vi "FSM_new.vi"() -> ()   [LabVIEW 2016]
panel:
  out "Current target":dbl[](array[numeric])
  out "note":string
  out "Waveform Graph 2":dbl[](graph)
  out "Select traing signal":i32
  out "Saved Target":dbl[][](array[numeric])
  out "Number of Signals":i32
  out "Signal Captured":dbl[][](array[numeric])
  in  "Signal Capture":bool
  out "Error_out":dbl[](array[numeric])
  out "Final Error":dbl
  out "Waveform Graph":dbl[](graph)
  in  "Inference":bool
  in  "Training":bool
  out "Enum":T1(ring)
  out "Weights_oX":dbl[][](array[numeric])
  out "Weights_hX":dbl[][](array[numeric])
  out "Outputs_oX":dbl[](array[numeric])
  out "Outputs_hX":dbl[](array[numeric])
  in  "Target 6":dbl
  in  "Target 5":dbl
  in  "Target 7":dbl
  in  "Target 8":dbl
  in  "Learning rate":dbl
  in  "Offset 2":dbl
  in  "Offset 1":dbl
  out "Random values generated":bool
  out "Training end":bool
  in  "A+E+F":dbl
  in  "A+B+D":dbl
  in  "C+Ch+B":dbl
  in  "C+E+G":dbl
  in  "Stop":bool
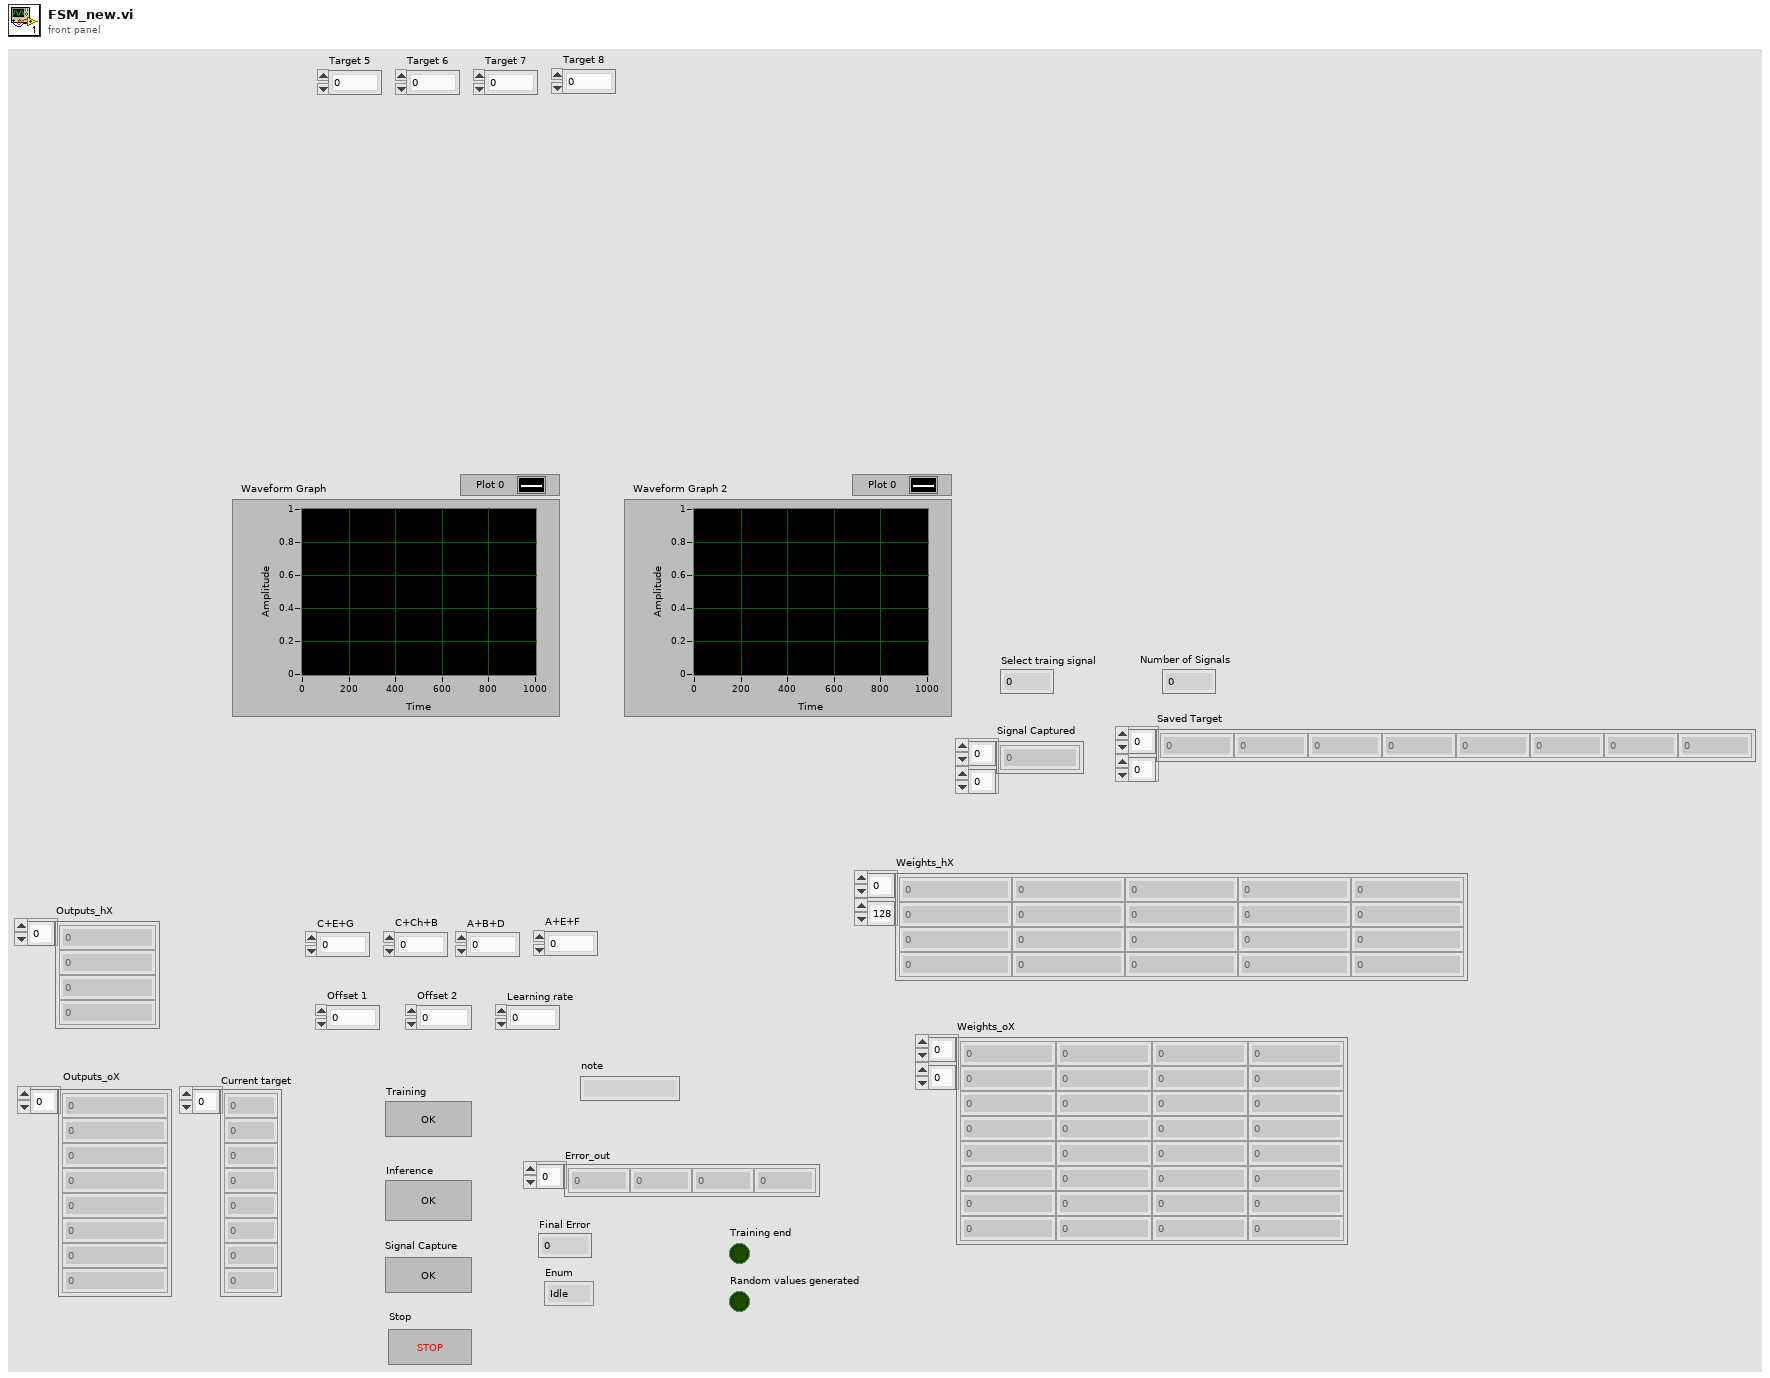
[diagram p1: front panel]
types:
  T1 = enum16{"Idle", "Generate weights", "Training mode", "Inference mode"}
  T2 = enum16{"Idle", "Generate weights", "Training mode", "Inference mode", "Signal Capture"}
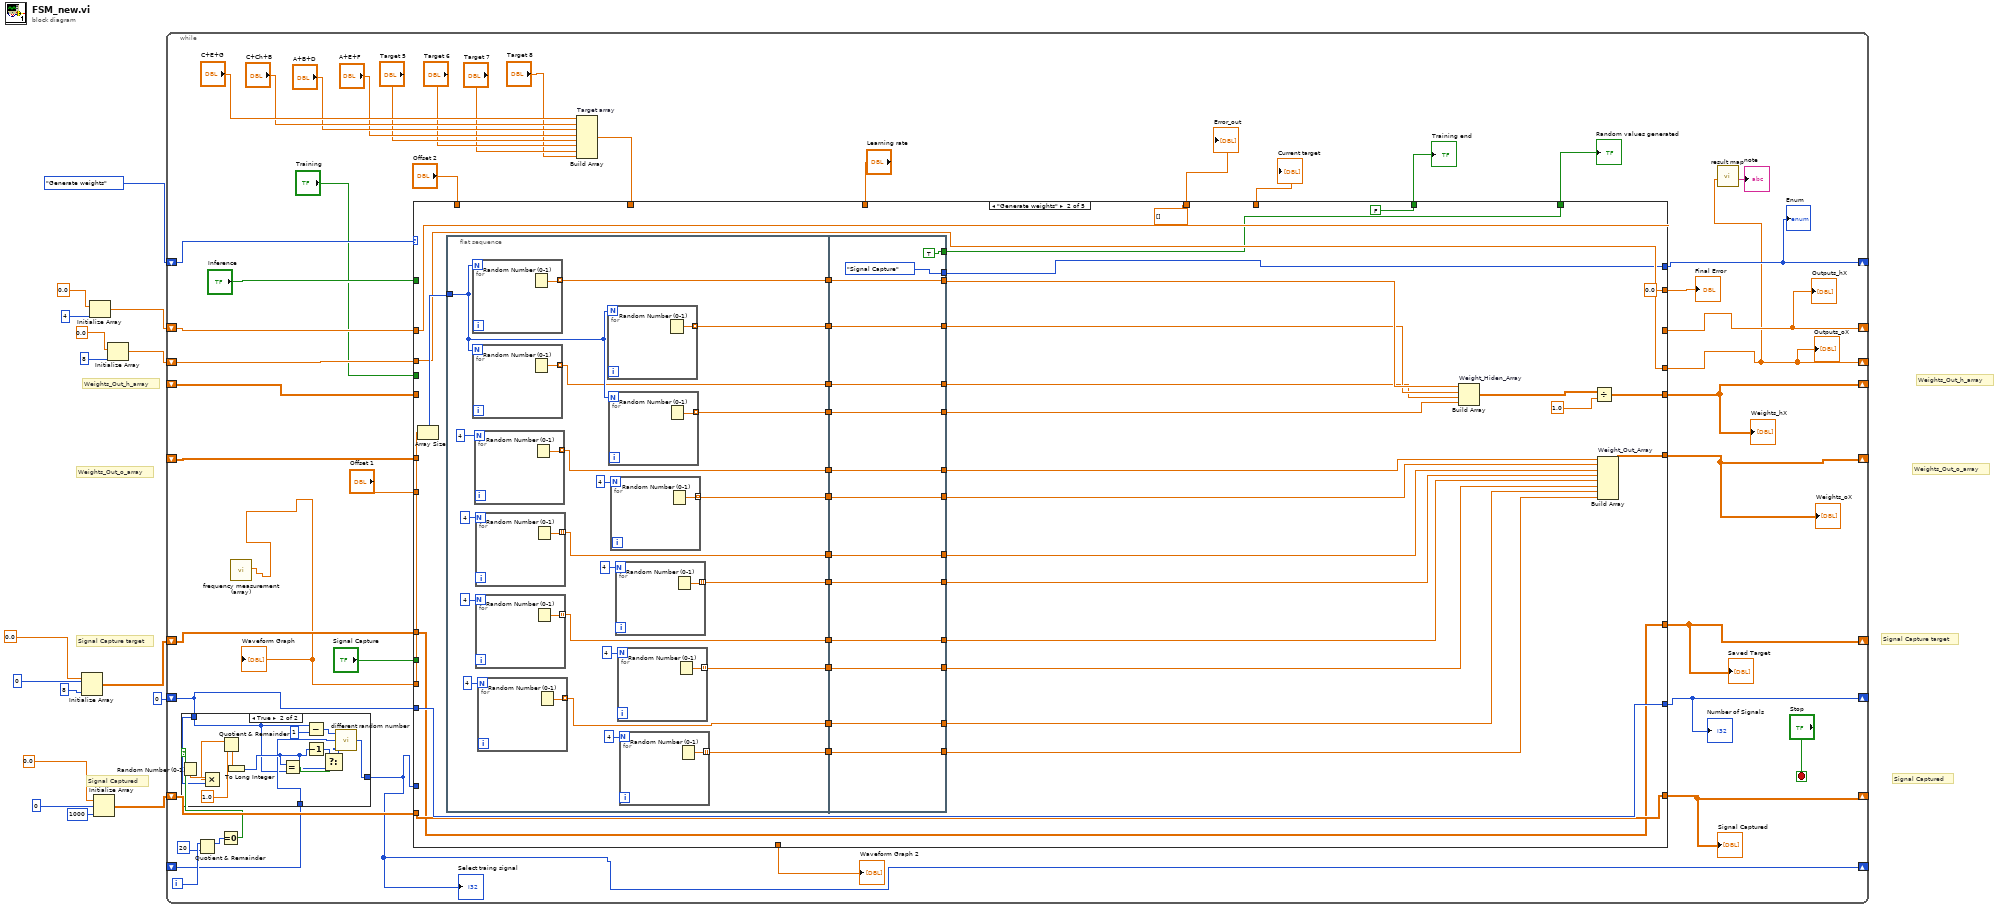
[diagram p0: block diagram]
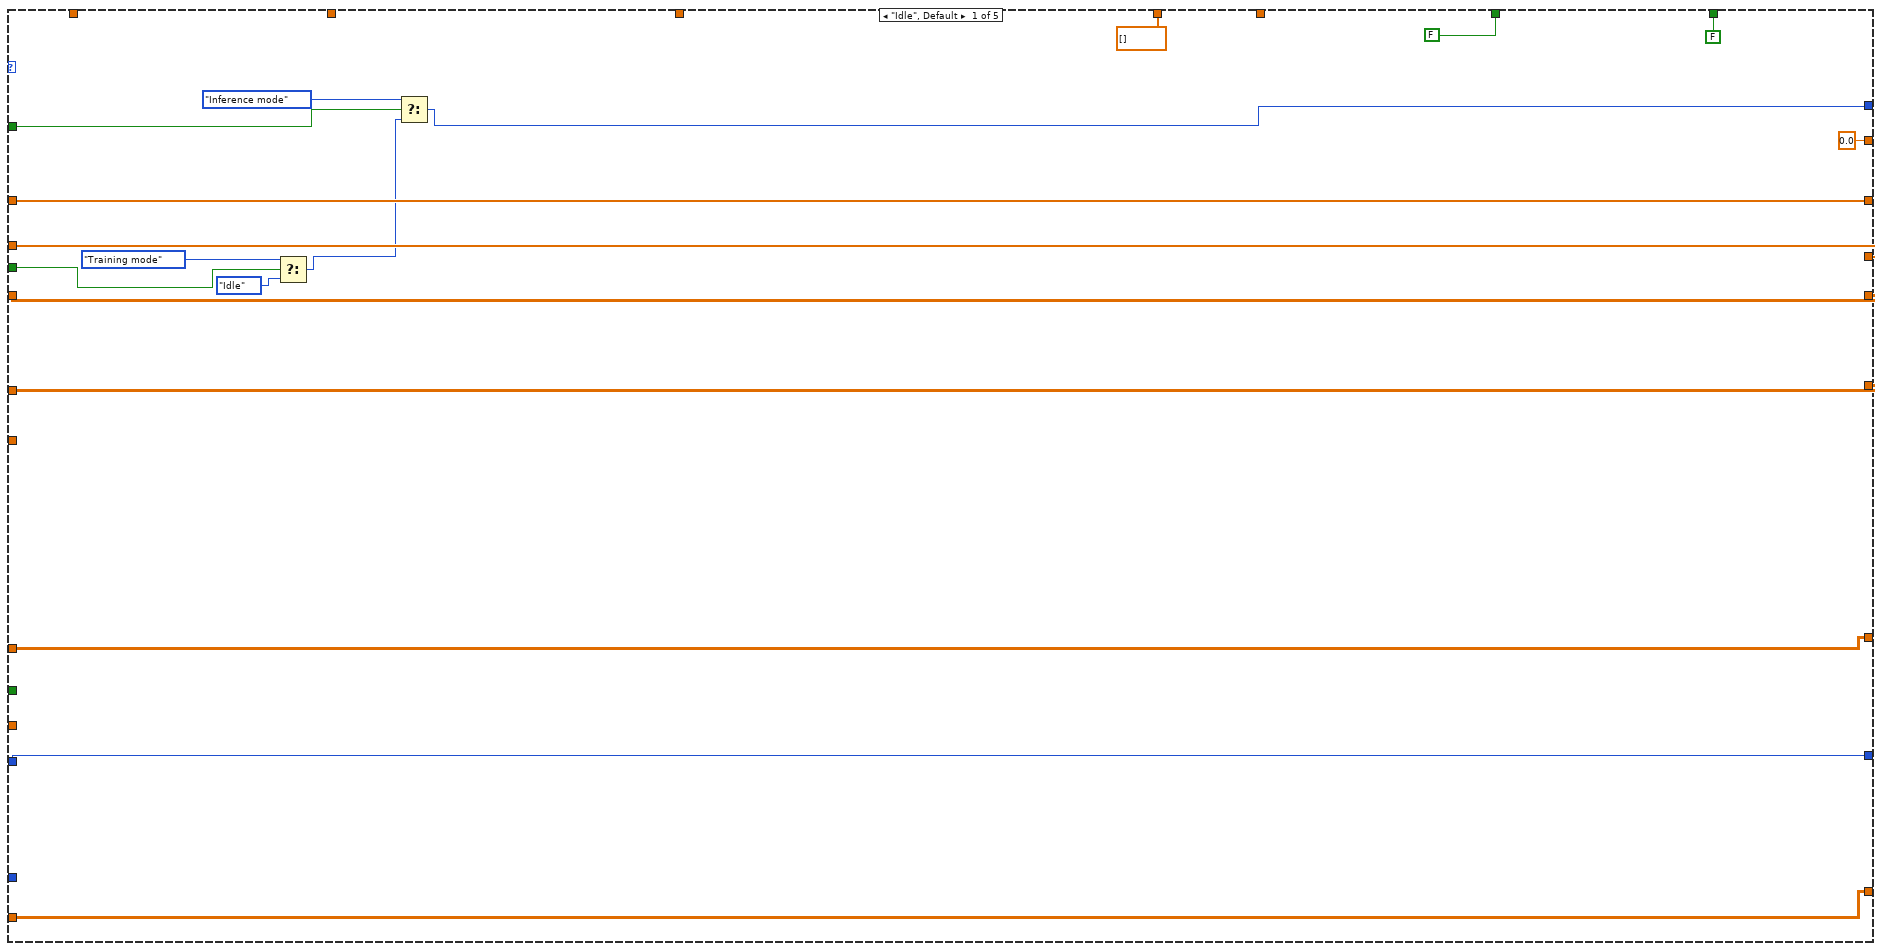
[diagram p3: hidden frame]
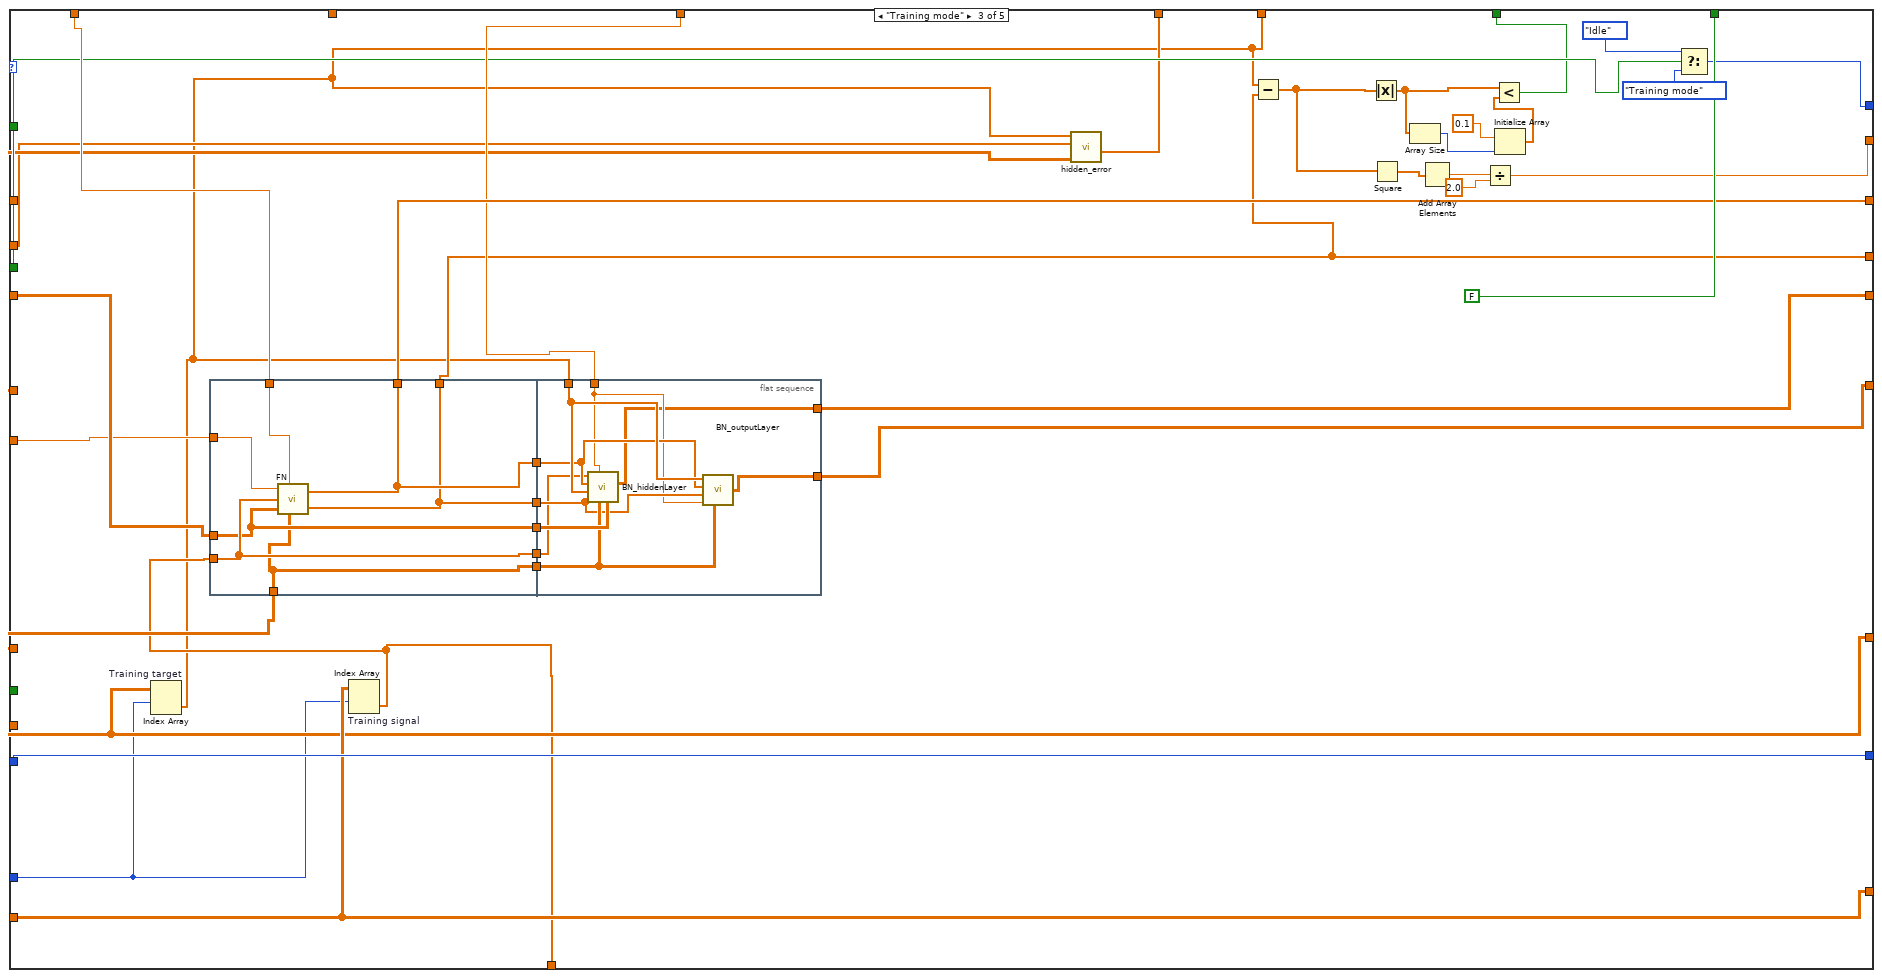
[diagram p4: hidden frame]
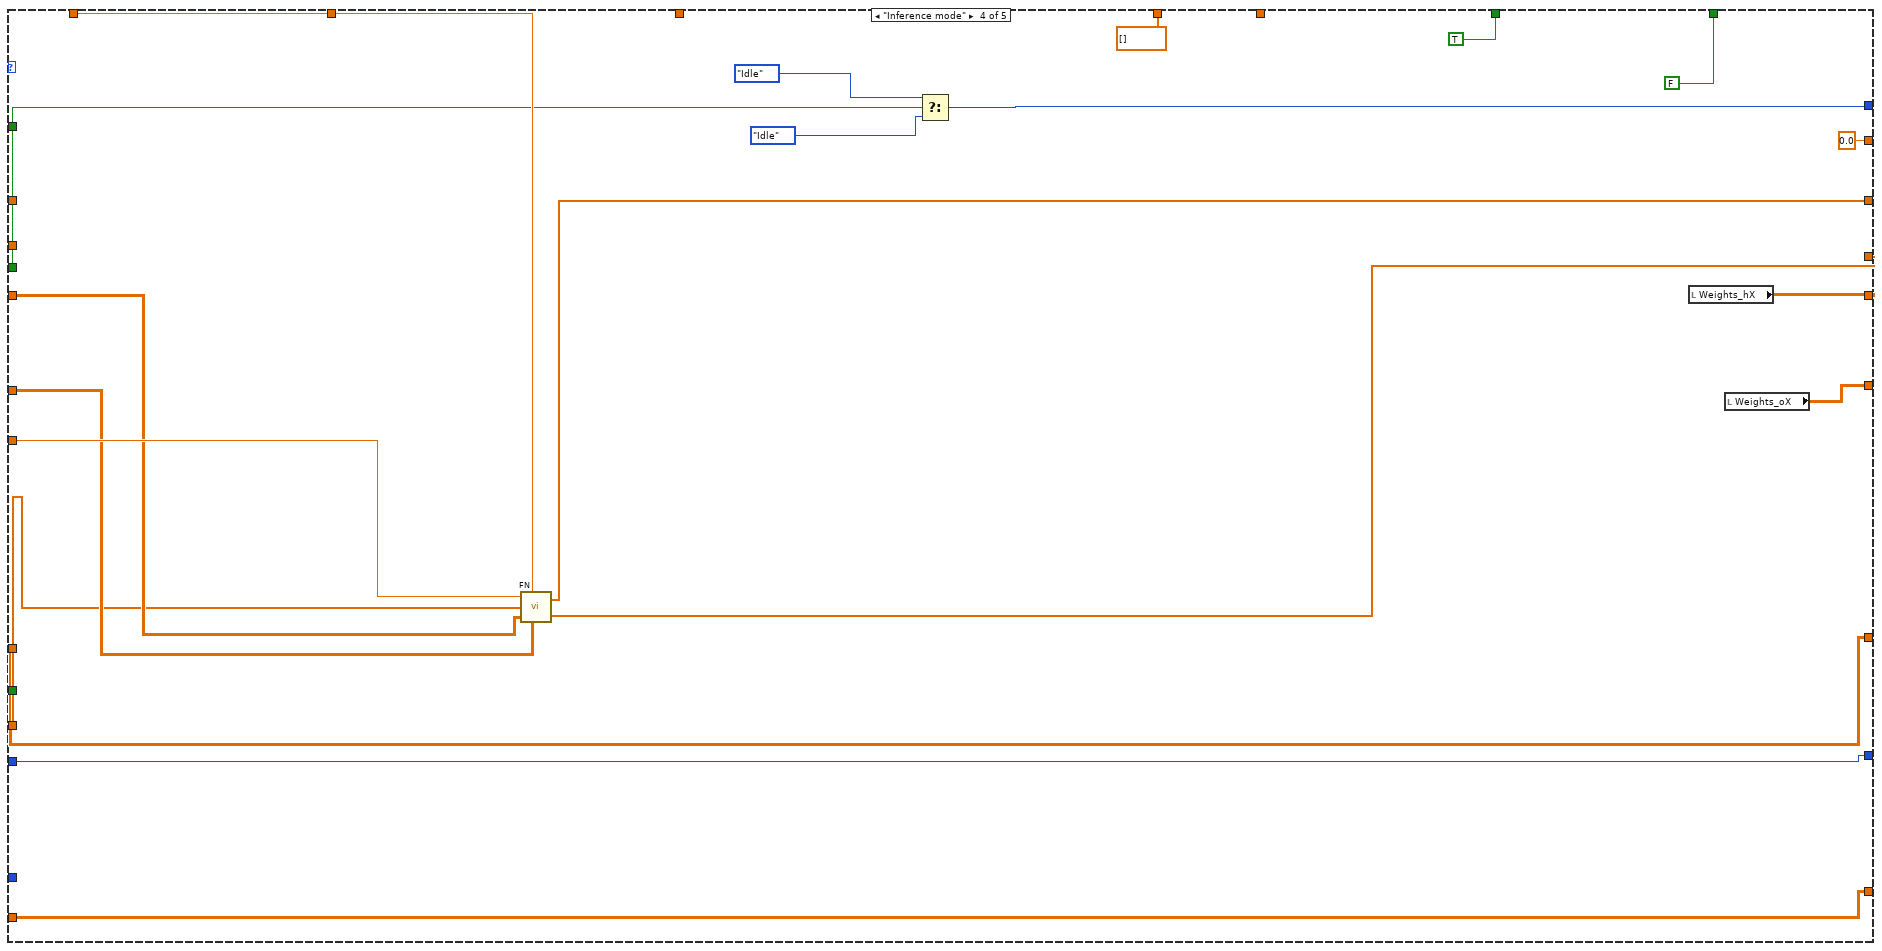
[diagram p5: hidden frame]
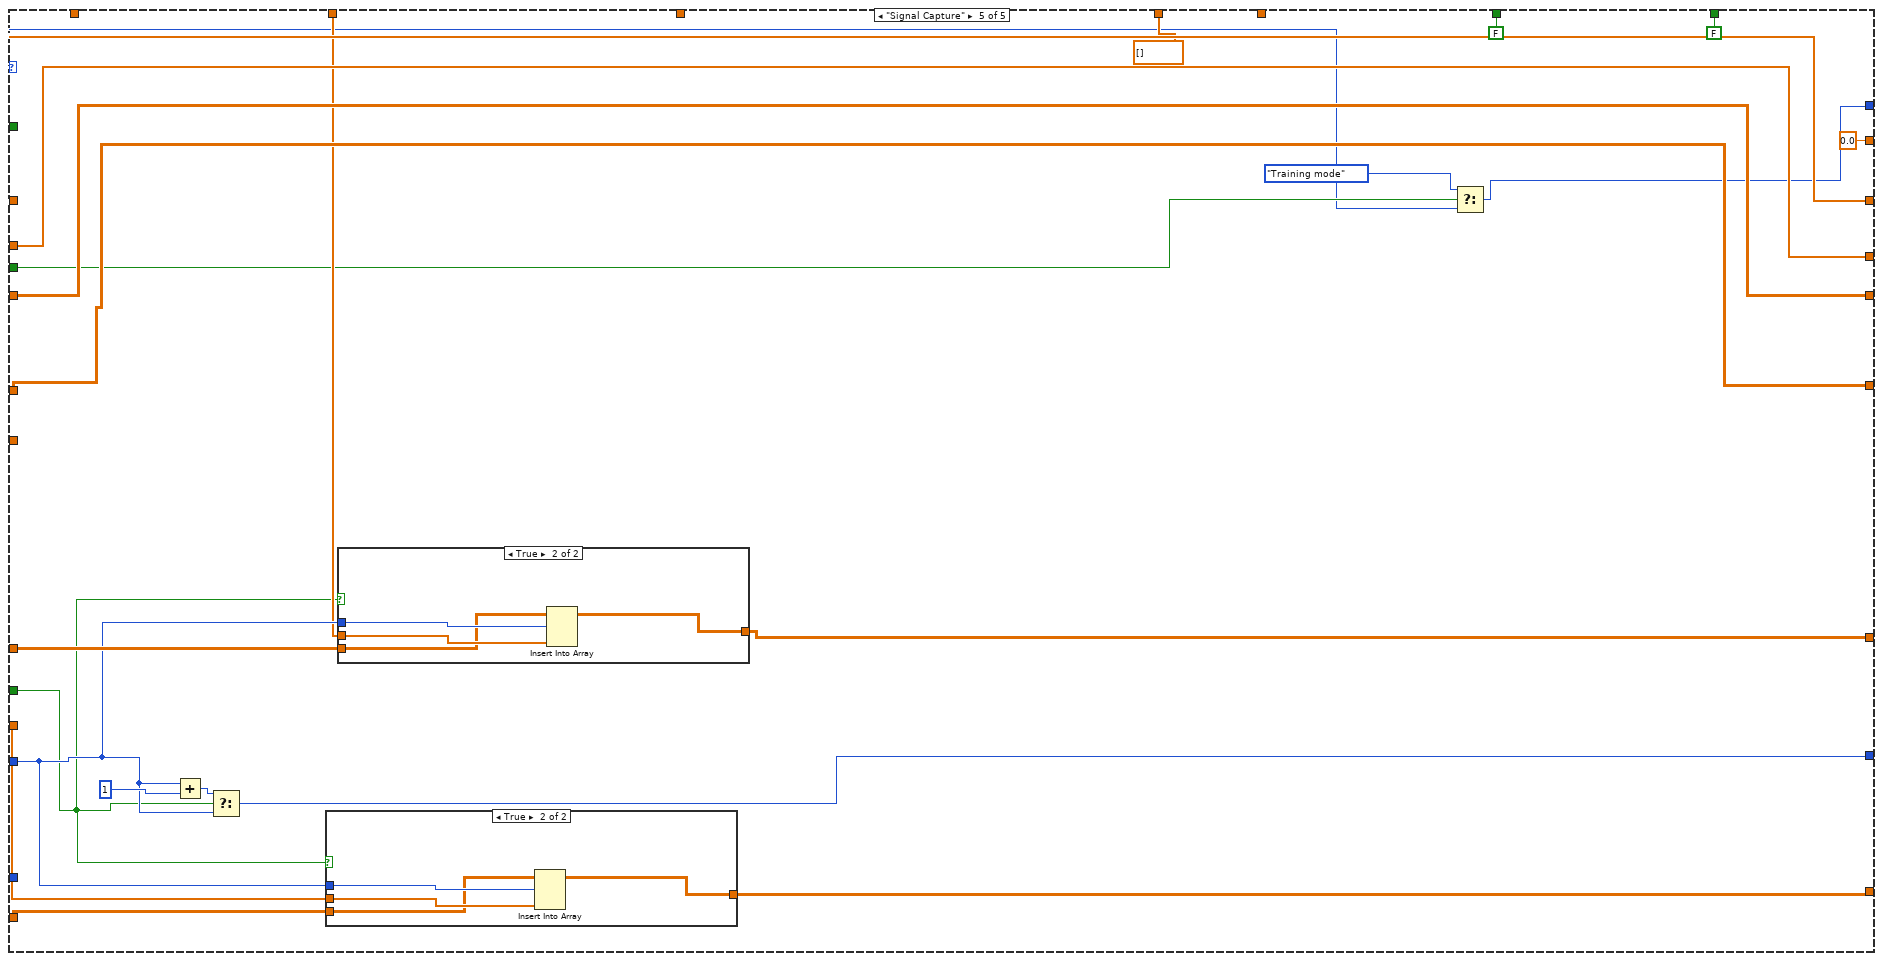
[diagram p6: hidden frame]
diagram:
  # "Signal Captured"
  # "Signal Capture target"
  # "Signal Captured"
  # "Signal Capture target"
  # "Weights_Out_o_array"
  # "Weights_Out_h_array"
  # "Weights_Out_o_array"
  # "Weights_Out_h_array"
  n1 = Initialize Array(0.0, 0, 8 ("dimension size")) -> (w1:dbl[][])
  n2 = Initialize Array(0.0, 4) -> (w15:dbl[])
  n3 = Initialize Array(0.0, 0, 1000 ("dimension size")) -> (w6:dbl[][])
  n4 = Initialize Array(0.0, 8) -> (w10:dbl[])
  n5 = while {
    shift-right: [w41] -> _
    shift-left: T2."Generate weights" -> [w58]
    shift-right: [w46] -> _
    shift-left: _ -> [w45]
    shift-right: [w47] -> _
    shift-left: _ -> [w44]
    shift-right: [w40] -> _
    shift-left: w15 -> [w43]
    shift-right: [w22] -> _
    shift-left: w10 -> [w42]
    shift-right: [w33] -> _
    shift-left: 0 -> [w19]
    shift-right: [w32] -> _
    shift-left: w6 -> [w31]
    shift-right: [w29] -> _
    shift-left: w1 -> [w30]
    shift-right: [w17] -> _
    shift-left: _ -> [w18]
    i -> [w26]
    stop <- "Stop" stop-if-true
    n6 = Quotient & Remainder(x=w26, y=20) -> (x-y*floor(x/y)=w24:i32)  [unwired: 1 out]
    n7 = Equal To 0?(x=w24) -> (x = 0?=w23:bool)
    n8 = case shown="True" w23 {
      tunnel: w19 -> [_ w65]
      tunnel: [w63 w69] -> w17
      tunnel: w18 -> [w63 w67]
      frame False {
      }
      frame True {
        n9 = Random Number (0-1)() -> (number: 0 to 1=w76:dbl)
        n10 = Multiply(x=w76, y=w65) -> (x*y=w75:dbl)
        n11 = Quotient & Remainder(x=w75, y=1.0) -> (floor(x/y)=w73:dbl)  [unwired: 1 out]
        n12 = To Long Integer(number=w73) -> (32bit integer=w70:i32)
        n13 = Equal?(x=w70, y=w65) -> (x = y?=w72:bool)
        n14 = Subtract(x=w65, y=1) -> (x-y=w66:i32)
        n15 = Decrement(x=w70) -> (x-1=w71:i32)
        n16 = Select(t=w71, s=w72, f=w70) -> (s? t:f=w68:i32)
        n17 = call "different random number.vi"("New one"=w68, "Last one"=w67, "Max"=w66) -> ("Final output"=w69:i32)
      }
    }
    "Select traing signal" <- w17
    n18 = call "frequency measurement (array).vi"() -> ("real part of fft array"=w27:dbl[])  [unwired: 11 in]
    "Waveform Graph" <- w27
    n19 = Build Array "Target array"("C+E+G", "C+Ch+B", "A+B+D", "A+E+F", "Target 5", "Target 6", "Target 7", "Target 8") -> (w49:dbl[])
    n20 = case shown="\"Generate weights\"" w58 {
      selector: w58 -> [_ _ _ _ w256]
      tunnel: [w82 w95 w204 w243 w258] -> w41
      tunnel: [FALSE w105 FALSE FALSE FALSE] -> w48
      tunnel: "Offset 1" -> [_ _ w216 w253 _]
      tunnel: "Offset 2" -> [_ _ w215 w254 _]
      tunnel: "Learning rate" -> [_ _ w213 _ _]
      tunnel: w49 -> [_ _ _ _ w261]
      tunnel: [w90 w108 w214 w252 w276] -> w40
      tunnel: [w89 w107 w207 w251 w275] -> w22
      tunnel: w27 -> [_ w106 _ w240 w266]
      tunnel: [w92 w102 w183 w249 w274] -> w46
      tunnel: [w91 w109 w199 w248 w273] -> w47
      tunnel: w45 -> [w92 _ w217 w247 w274]
      tunnel: w44 -> [w91 _ w191 w246 w273]
      tunnel: w43 -> [w90 w108 _ _ w276]
      tunnel: w42 -> [w89 w107 w190 _ w275]
      tunnel: "Training" -> [w87 _ w198 w242 w257]
      tunnel: [FALSE FALSE w197 TRUE FALSE] -> w39
      tunnel: "Inference" -> [w84 _ _ _ _]
      tunnel: [0.0 0.0 w192 0.0 0.0] -> w36
      tunnel: [dbl[] [] ("Error_out") dbl[] [] ("Error_out") w189 dbl[] [] ("Error_out") dbl[] [] ("Error_out")] -> w35
      tunnel: "Signal Capture" -> [_ _ _ _ w260]
      tunnel: [w78 w98 w188 w237 w267] -> w33
      tunnel: w19 -> [w78 w98 w188 w237 w262]
      tunnel: [w79 w97 w187 w236 w265] -> w32
      tunnel: w31 -> [w79 w97 w187 w236 w264]
      tunnel: w30 -> [w77 w96 w186 w235 w263]
      tunnel: [w77 w96 w186 w235 w259] -> w29
      tunnel: w17 -> [_ _ w184 _ _]
      tunnel: [_ _ w185 _ _] -> w28
      tunnel: [_ _ w182 _ _] -> w20
      frame "Idle", Default {
        n21 = Select(t=T1."Training mode", s=w87, f=T1."Idle") -> (s? t:f=w83:T1)
        n22 = Select(t=T1."Inference mode", s=w84, f=w83) -> (s? t:f=w82:T1)
      }
      frame "Generate weights" {
        n23 = Array Size(array=w106) -> (size(s)=w134:i32)
        n24 = flat-sequence {
          tunnel: w134 -> [w155]
          tunnel: [w154] -> w133
          tunnel: [w153] -> w132
          tunnel: [w152] -> w131
          tunnel: [w151] -> w130
          tunnel: [w150] -> w129
          tunnel: [w149] -> w128
          tunnel: [w148] -> w127
          tunnel: [w147] -> w126
          tunnel: [w146] -> w125
          tunnel: [w145] -> w124
          tunnel: [w144] -> w123
          tunnel: [w143] -> w122
          tunnel: [TRUE] -> w105
          tunnel: w133 -> [w180]
          tunnel: [w180] -> w121
          tunnel: w132 -> [w179]
          tunnel: [w179] -> w119
          tunnel: w131 -> [w178]
          tunnel: [w178] -> w110
          tunnel: w130 -> [w177]
          tunnel: [w177] -> w112
          tunnel: w129 -> [w176]
          tunnel: [w176] -> w114
          tunnel: w128 -> [w175]
          tunnel: [w175] -> w116
          tunnel: w127 -> [w174]
          tunnel: [w174] -> w120
          tunnel: w126 -> [w173]
          tunnel: [w173] -> w118
          tunnel: w125 -> [w172]
          tunnel: [w172] -> w111
          tunnel: w124 -> [w171]
          tunnel: [w171] -> w113
          tunnel: [w170] -> w115
          tunnel: w123 -> [w170]
          tunnel: w122 -> [w169]
          tunnel: [w169] -> w117
          tunnel: [T2."Signal Capture"] -> w95
          frame #0 {
            n25 = for {
              N: w155 -> [_]
              tunnel: [w167] -> w154 mode=indexing
              n26 = Random Number (0-1)() -> (number: 0 to 1=w167:dbl)
            }
            n27 = for {
              N: w155 -> [_]
              tunnel: [w166] -> w153 mode=indexing
              n28 = Random Number (0-1)() -> (number: 0 to 1=w166:dbl)
            }
            n29 = for {
              N: 4 -> [_]
              tunnel: [w165] -> w152 mode=indexing
              n30 = Random Number (0-1)() -> (number: 0 to 1=w165:dbl)
            }
            n31 = for {
              N: 4 -> [_]
              tunnel: [w161] -> w151 mode=indexing
              n32 = Random Number (0-1)() -> (number: 0 to 1=w161:dbl)
            }
            n33 = for {
              N: 4 -> [_]
              tunnel: [w163] -> w150 mode=indexing
              n34 = Random Number (0-1)() -> (number: 0 to 1=w163:dbl)
            }
            n35 = for {
              N: 4 -> [_]
              tunnel: [w164] -> w149 mode=indexing
              n36 = Random Number (0-1)() -> (number: 0 to 1=w164:dbl)
            }
            n37 = for {
              N: w155 -> [_]
              tunnel: [w162] -> w148 mode=indexing
              n38 = Random Number (0-1)() -> (number: 0 to 1=w162:dbl)
            }
            n39 = for {
              N: w155 -> [_]
              tunnel: [w160] -> w147 mode=indexing
              n40 = Random Number (0-1)() -> (number: 0 to 1=w160:dbl)
            }
            n41 = for {
              N: 4 -> [_]
              tunnel: [w159] -> w146 mode=indexing
              n42 = Random Number (0-1)() -> (number: 0 to 1=w159:dbl)
            }
            n43 = for {
              N: 4 -> [_]
              tunnel: [w158] -> w145 mode=indexing
              n44 = Random Number (0-1)() -> (number: 0 to 1=w158:dbl)
            }
            n45 = for {
              N: 4 -> [_]
              tunnel: [w157] -> w144 mode=indexing
              n46 = Random Number (0-1)() -> (number: 0 to 1=w157:dbl)
            }
            n47 = for {
              N: 4 -> [_]
              tunnel: [w156] -> w143 mode=indexing
              n48 = Random Number (0-1)() -> (number: 0 to 1=w156:dbl)
            }
          }
          frame #1 {
          }
        }
        n49 = Build Array "Weight_Hiden_Array"(w121, w120, w119, w118) -> (w103:dbl[][])
        n50 = Divide(x=w103, y=1.0) -> (x/y=w102:dbl[][])
        n51 = Build Array "Weight_Out_Array"(w110, w111, w112, w113, w114, w115, w116, w117) -> (w109:dbl[][])
      }
      frame "Training mode" {
        n52 = Index Array "Training target"(array=w186, index (row)=w184) -> (element=w182:dbl[])  [unwired: 1 in]
        n53 = flat-sequence {
          tunnel: w185 -> [w223]
          tunnel: w217 -> [w221]
          tunnel: w191 -> [w220]
          tunnel: w216 -> [w225]
          tunnel: w215 -> [w224]
          tunnel: [w222] -> w214
          tunnel: [w219] -> w207
          tunnel: [w223] -> w212
          tunnel: [w222] -> w211
          tunnel: [w219] -> w210
          tunnel: [w221] -> w209
          tunnel: [w220] -> w208
          tunnel: w213 -> [w227]
          tunnel: [w234] -> w199
          tunnel: w212 -> [w228]
          tunnel: w211 -> [w229]
          tunnel: w182 -> [w230]
          tunnel: w210 -> [w231]
          tunnel: w209 -> [w233]
          tunnel: w208 -> [w232]
          tunnel: [w226] -> w183
          frame #0 {
            n54 = call "FN.vi"("Offset_h"=w225, "Offset_out"=w224, "Inputs"=w223, "Weights_h"=w221, "Weights_out"=w220) -> ("Outputs_hx"=w222:dbl[], "Outputs_out"=w219:dbl[])
          }
          frame #1 {
            n55 = call "BN_hiddenLayer.vi"("Weights_hX_IN"=w233, "Weights_outX(before being updated)"=w232, "Learning rate"=w227, "Out_outX"=w231, "Target_outX"=w230, "Out_hx"=w229, "Inputs"=w228) -> ("Weights_hX_OUT"=w226:dbl[][])  [unwired: 3 in]
            n56 = call "BN_outputLayer.vi"("Target_outX"=w230, "Out_hx"=w229, "Out_outX"=w231, "Learning rate"=w227, "Weights_outX_IN"=w232) -> ("Weights_outX_OUT"=w234:dbl[][])
          }
        }
        n57 = Index Array "Training signal"(array=w187, index (row)=w184) -> (element=w185:dbl[])  [unwired: 1 in]
        n58 = call "hidden_error.vi"("Weight"=w191, "Output"=w190, "Target"=w182) -> ("Error_out"=w189:dbl[])  [unwired: 8 in]
        n59 = Subtract(x=w182, y=w207) -> (x-y=w196:dbl[])
        n60 = Absolute Value(x=w196) -> (abs(x)=w202:dbl[])
        n61 = Square(x=w196) -> (x^2=w195:dbl[])
        n62 = Array Size(array=w202) -> (size(s)=w201:i32)
        n63 = Add Array Elements(numeric array=w195) -> (sum=w194:dbl)
        n64 = Divide(x=w194, y=2.0) -> (x/y=w192:dbl)
        n65 = Initialize Array(0.1 ("y"), w201) -> (w200:dbl[])
        n66 = Less?(x=w202, y=w200) -> (x < y?=w197:bool)
        n67 = Select(t=T1."Idle", s=w198, f=T1."Training mode") -> (s? t:f=w204:T1)
      }
      frame "Inference mode" {
        n68 = call "FN.vi"("Offset_h"=w253, "Offset_out"=w254, "Inputs"=w240, "Weights_h"=w247, "Weights_out"=w246) -> ("Outputs_hx"=w252:dbl[], "Outputs_out"=w251:dbl[])
        n69 = Select(t=T1."Idle", s=w242, f=T1."Idle") -> (s? t:f=w243:T1)
        n70 = local read "Weights_hX"() -> (w249:dbl[][])
        n71 = local read "Weights_oX"() -> (w248:dbl[][])
      }
      frame "Signal Capture" {
        n72 = Add(x=w262, y=1) -> (x+y=w269:i32)
        n73 = Select(t=w269, s=w260, f=w262) -> (s? t:f=w267:i32)
        n74 = case shown="True" w260 {
          tunnel: w262 -> [_ w287]
          tunnel: w266 -> [_ w286]
          tunnel: [w283 w285] -> w265
          tunnel: w264 -> [w283 w284]
          frame False {
          }
          frame True {
            n75 = Insert Into Array(array=w284, index (row)=w287, new element=w286) -> (w285:dbl[][])  [unwired: 1 in]
          }
        }
        n76 = case shown="True" w260 {
          tunnel: w262 -> [_ w282]
          tunnel: w261 -> [_ w281]
          tunnel: [w278 w280] -> w259
          tunnel: w263 -> [w278 w279]
          frame False {
          }
          frame True {
            n77 = Insert Into Array(array=w279, index (row)=w282, new element=w281) -> (w280:dbl[][])  [unwired: 1 in]
          }
        }
        n78 = Select(t=T2."Training mode", s=w257, f=w256) -> (s? t:f=w258:T2)
      }
    }
    "Weights_hX" <- w46
    "Weights_oX" <- w47
    "Random values generated" <- w48
    "Enum" <- w41
    "Outputs_hX" <- w40
    "Outputs_oX" <- w22
    "Training end" <- w39
    "Final Error" <- w36
    "Error_out" <- w35
    "Number of Signals" <- w33
    "Signal Captured" <- w32
    "Saved Target" <- w29
    "Waveform Graph 2" <- w28
    "Current target" <- w20
    n79 = call "result map.vi"("output"=w22) -> ("note"=→"note":string)  [unwired: 10 in]
  }
